vi "AbortTrial.vi"(8 "error in (no error)":errorcluster, 10 "AbortReason":string, 11 "TrialBasedExperiment in":refnum<class "TrialBasedExperiment.lvclass">) -> (0 "error out":errorcluster, 3 "TrialBasedExperiment out":refnum<class "TrialBasedExperiment.lvclass">)   [LabVIEW 2012, in "AcquisitionCoreObjects.lvlib" / "TrialBasedExperiment.lvclass"]
uses:
  TrialBasedExperiment.lvclass
  TrialBasedExperiment.lvclass/TrialBasedExperiment.ctl
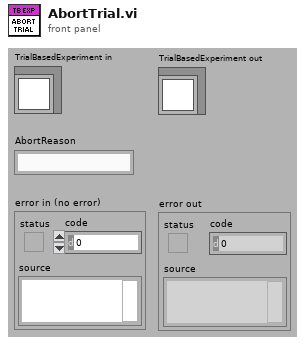
[diagram p1: front panel]
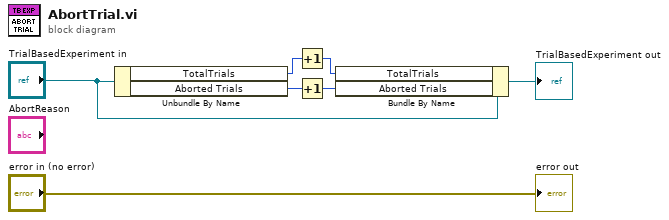
[diagram p0: block diagram]
diagram:
  n1 = Unbundle By Name("TrialBasedExperiment in") -> ("TotalTrials"=w4:u32, "Aborted Trials"=w6:u32)
  n2 = Increment(x=w4) -> (x+1=w3:u32)
  n3 = Increment(x=w6) -> (x+1=w5:u32)
  n4 = Bundle By Name(cluster="TrialBasedExperiment in", "TotalTrials"=w3, "Aborted Trials"=w5) -> (→"TrialBasedExperiment out":refnum<class "TrialBasedExperiment.lvclass">)
  "error out" <- "error in (no error)"
